vi "Get Control Refnums by Names.vi"(8 "error in":errorcluster, 9 "Selection":T1(ring), 10 "Control Labels":string[](array[string]), 11 "VI  Ref":refnum<vi>) -> (0 "error out":errorcluster, 1 "All Ctls found?":bool, 2 "Ctl Refnums":refnum<vi>[](array[refnum]), 3 "VI  Ref (out)":refnum<vi>)   [LabVIEW 2019]
doc: "Returns an array of control refnums, labels and data, from the front panel of the calling VI.\n\nThis VI also accounts for tab controls within other tab controls."
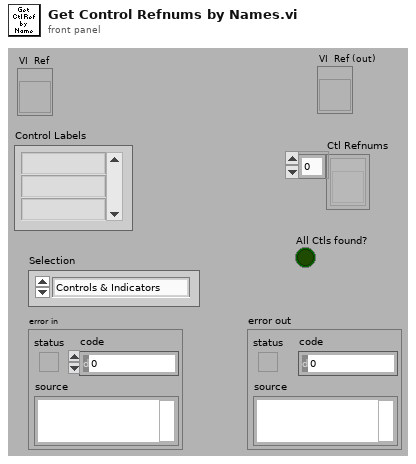
[diagram p1: front panel]
types:
  T1 = enum16{"Controls & Indicators", "Controls", "Indicators"}
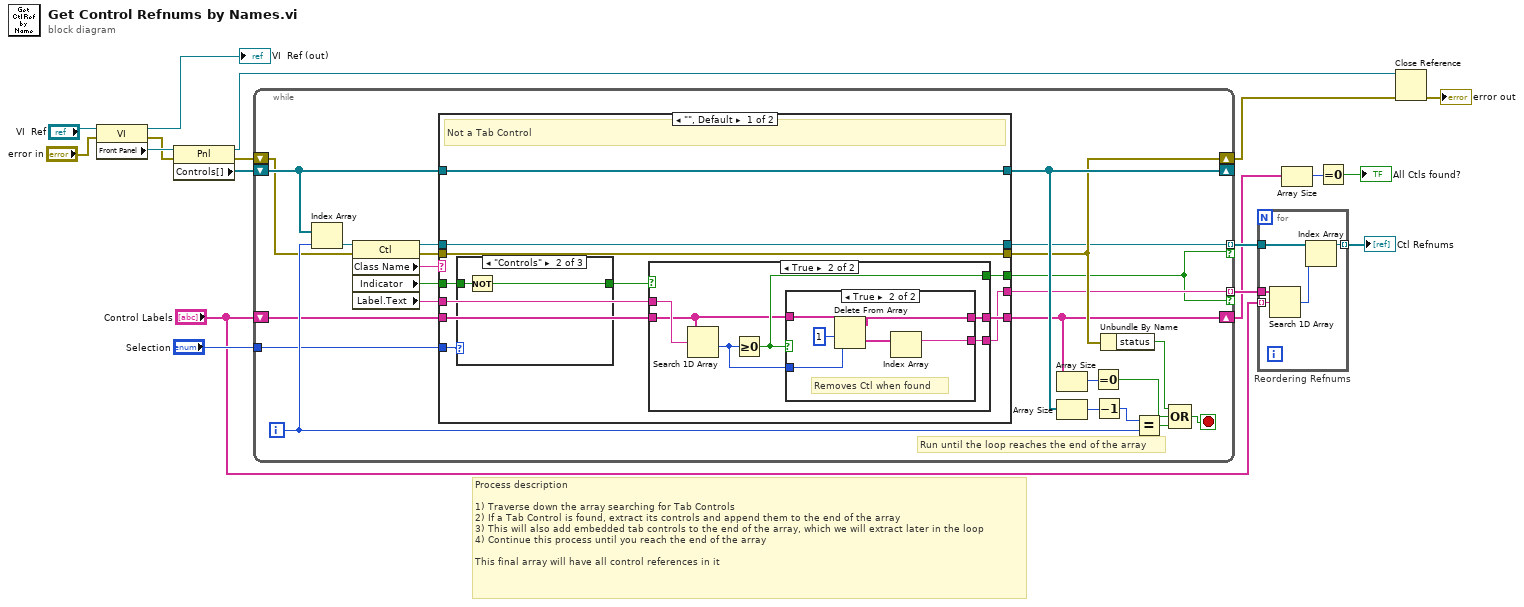
[diagram p0: block diagram]
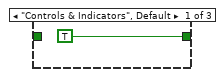
[diagram p4: hidden frame]
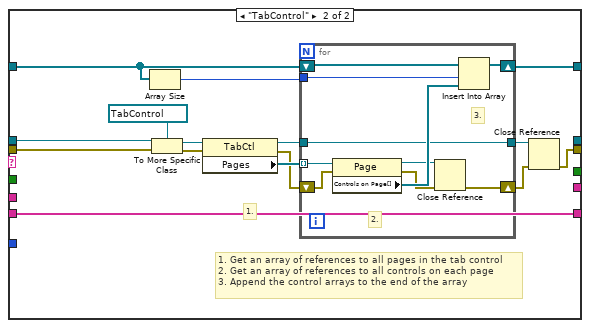
[diagram p6: hidden frame]
diagram:
  # "Process description\n\n1) Traverse down the array searching for Tab Controls\n2) If a Tab Control is found, extract its controls and append them to the end of the array\n3) This will also add embedded tab controls to the end of the array, which we will extract later in the loop\n4) Continue this process until you reach the end of the array\n\nThis final array will have all control references in it"
  n1 = property class="VI"(reference="VI  Ref", error in="error in") -> (reference out=→"VI  Ref (out)":refnum<vi>, error out=w16:errorcluster, "Front Panel"=w17:refnum<vi>)
  n2 = property class="Pnl"(reference=w17, error in=w16) -> (reference out=w14:refnum<vi>, error out=w15:errorcluster, "Controls[]"=w18:refnum<vi>[])
  n3 = while {
    shift-right: [w35] -> _
    shift-left: w18 -> [w41]
    shift-right: [w32] -> w13
    shift-left: w15 -> [w34]
    shift-right: [w25] -> w1
    shift-left: "Control Labels" -> [w27]
    tunnel: [w26] -> w5 mode=indexing if=w19
    tunnel: "Selection" -> [w21]
    tunnel: [w20] -> w2 mode=indexing if=w19
    i -> [w36]
    stop <- w30 stop-if-true
    # "Run until the loop reaches the end of the array"
    n4 = Index Array(array=w41, index=w36) -> (element=w37:refnum<vi>)
    n5 = property class="Ctl"(reference=w37, error in=w34) -> (reference out=w42:refnum<vi>, error out=w33:errorcluster, "Class Name"=w40:string, "Indicator"=w22:bool, "Label.Text"=w28:string)
    n6 = case shown="\"\", Default" w40 {
      tunnel: w42 -> [w50 w86]
      tunnel: w41 -> [w53 w82]
      tunnel: [w53 w83] -> w35
      tunnel: w33 -> [w52 w79]
      tunnel: [w52 w75] -> w32
      tunnel: w28 -> [w51 _]
      tunnel: w27 -> [w48 w72]
      tunnel: [w50 _] -> w26
      tunnel: [w49 _] -> w19
      tunnel: [w47 w72] -> w25
      tunnel: w22 -> [w45 _]
      tunnel: w21 -> [w46 _]
      tunnel: [w43 _] -> w20
      frame "", Default {
        # "Not a Tab Control"
        n7 = case shown="\"Controls\"" w46 {
          tunnel: w45 -> [_ w70 w71]
          tunnel: [TRUE ("Indicator") w69 w71] -> w44
          frame "Controls & Indicators", Default {
          }
          frame "Controls" {
            n8 = Not(x=w70) -> (.not. x?=w69:bool)
          }
          frame "Indicators" {
          }
        }
        n9 = case shown="True" w44 {
          tunnel: w51 -> [_ w60]
          tunnel: [_ w59] -> w49
          tunnel: w48 -> [w54 w58]
          tunnel: [w54 w56] -> w47
          tunnel: [_ w55] -> w43
          frame False {
          }
          frame True {
            n10 = Search 1D Array(1D array=w58, element=w60) -> (index of element=w57:i32)  [unwired: 1 in]
            n11 = Greater Or Equal To 0?(x=w57) -> (x >= 0?=w59:bool)
            n12 = case shown="True" w59 {
              tunnel: w58 -> [w61 w67]
              tunnel: w57 -> [_ w66]
              tunnel: [w61 w64] -> w56
              tunnel: [_ w62] -> w55
              frame False {
              }
              frame True {
                # "Removes Ctl when found"
                n13 = Delete From Array(array=w67, length=1, index=w66) -> (deleted portion=w63:string[], array with subset deleted=w64:string[])
                n14 = Index Array(array=w63) -> (element=w62:string)  [unwired: 1 in]
              }
            }
          }
        }
      }
      frame "TabControl" {
        # "1. Get an array of references to all pages in the tab control\n2. Get an array of references to all controls on each page\n3. Append the control arrays to the end of the array"
        # "1."
        n15 = Array Size(array=w82) -> (size(s)=w80:i32)
        n16 = To More Specific Class(target class=refnum<vi> refnum ("Tab Control"), reference=w86, error in=w79) -> (specific class reference=w85:refnum<vi>, error out=w78:errorcluster)
        n17 = property class="TabCtl"(reference=w85, error in=w78) -> (reference out=w76:refnum<vi>, error out=w77:errorcluster, "Pages"=w84:refnum<vi>[])
        n18 = for {
          tunnel: w84 -> [w96] mode=indexing
          tunnel: w80 -> [w94]
          shift-right: [w95] -> w83
          shift-left: w82 -> [w93]
          tunnel: w76 -> [w90]
          tunnel: [w90] -> w74
          shift-right: [w87] -> w73
          shift-left: w77 -> [w91]
          # "3."
          # "2."
          n19 = property class="Page"(reference=w96, error in=w91) -> (reference out=w89:refnum<vi>, error out=w88:errorcluster, "Controls on Page[]"=w92:refnum<vi>[])
          n20 = Close Reference(reference=w89, error in (no error)=w88) -> (error out=w87:errorcluster)
          n21 = Insert Into Array(array=w93, index=w94, new element=w92) -> (w95:refnum<vi>[])
        }
        n22 = Close Reference(reference=w74, error in (no error)=w73) -> (error out=w75:errorcluster)
      }
    }
    n23 = Array Size(array=w25) -> (size(s)=w24:i32)
    n24 = Array Size(array=w35) -> (size(s)=w39:i32)
    n25 = Equal To 0?(x=w24) -> (x = 0?=w23:bool)
    n26 = Decrement(x=w39) -> (x-1=w38:i32)
    n27 = Unbundle By Name(w32) -> ("status"=w29:bool)
    n28 = Equal?(x=w38, y=w36) -> (x = y?=w31:bool)
    n29 = Compound Arithmetic op=OR(w29, w23, w31) -> (w30:bool)
  }
  n30 = for "Reordering Refnums" {
    tunnel: w5 -> [w101]
    tunnel: [w99] -> w4 mode=indexing
    tunnel: "Control Labels" -> [w98] mode=indexing
    tunnel: w2 -> [w97]
    n31 = Search 1D Array(1D array=w97, element=w98) -> (index of element=w100:i32)  [unwired: 1 in]
    n32 = Index Array(array=w101, index=w100) -> (element=w99:refnum<vi>)
  }
  "Ctl Refnums" <- w4
  n33 = Array Size(array=w1) -> (size(s)=w8:i32)
  n34 = Equal To 0?(x=w8) -> (x = 0?=→"All Ctls found?":bool)
  n35 = Close Reference(reference=w14, error in (no error)=w13) -> (error out=→"error out":errorcluster)
